vi "课堂.vi"() -> ()   [LabVIEW 2025]
panel:
  out "波形图表 7":dynamicdata(graph)
  out "波形图 4":cluster{dbl, dbl, dbl[]}[](graph)
  out "波形图表 6":dynamicdata(graph)
  out "波形图表 5":dbl[][](graph)
  out "波形图表 4":dbl[][](graph)
  out "波形图表 3":T1(graph)
  in  "数值":i32=40
  out "波形图表 2":dbl(graph)
  out "添加的数组":cluster{dbl[], dbl, dbl}[](array[cluster])
  out "波形图表":dbl[](graph)
  out "波形图 3":cluster{dbl[]}[](graph)
  out "波形图 2":dbl[][](graph)
  in  "采样点":i32=20
  out "波形图":dbl[](graph)=[0.8868508827682611, 0.2984304319078226, 0.11493741001008173, 0.9364201331616009, 0.9408037968299381, 0.6329733796655734, 0.6472915833351531, 0.9860727906146628, 0.3603313120178604, 0.38096386458152054, 0.8470946380077311, 0.620762260365446, 0.1766664398823562, 0.1967040576165764, 0.5080598419098434, 0.6274260346713301, 0.000348958293627355, 0.6443450592231559, 0.20809398466731732, 0.32035543006157274]
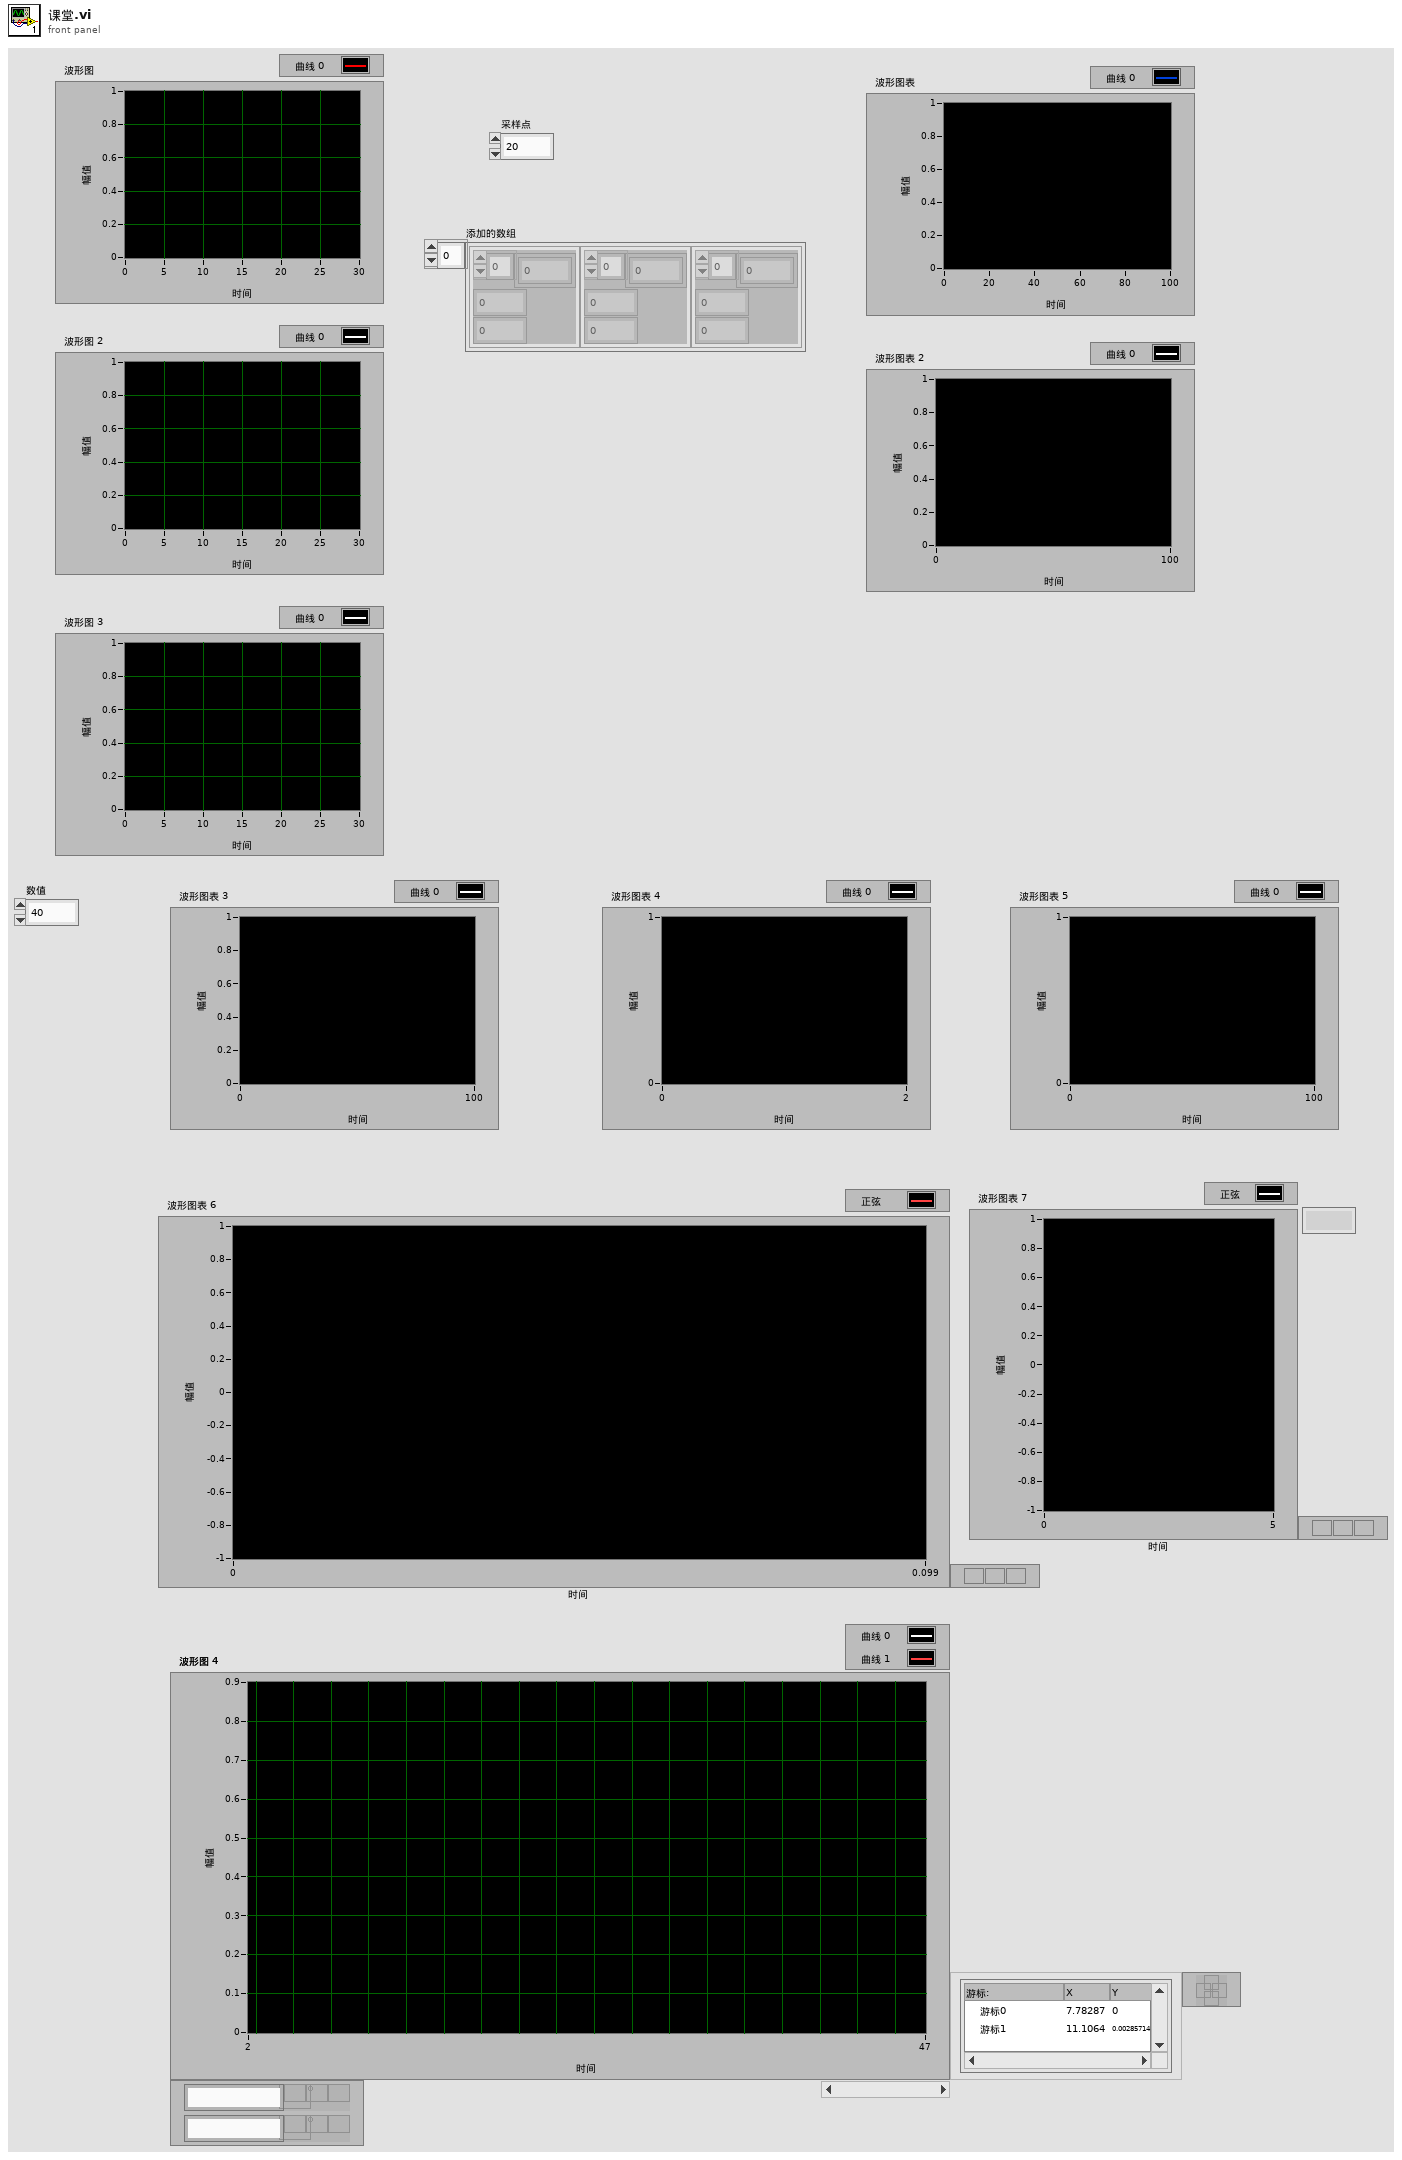
[diagram p1: front panel]
types:
  T1 = cluster{"number: 0 to 1":dbl, "number: 0 to 1":dbl}
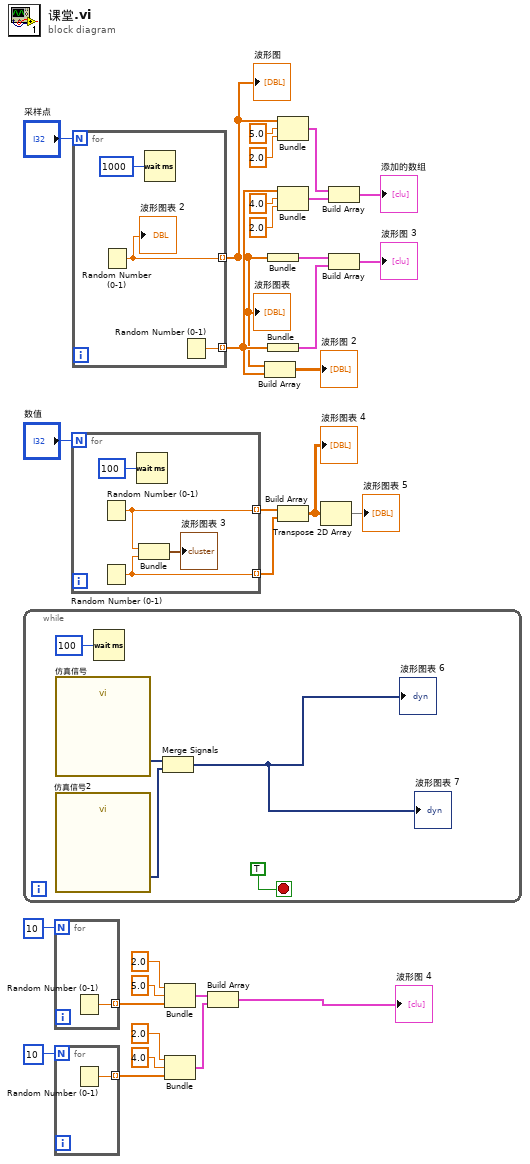
[diagram p0: block diagram]
diagram:
  n1 = while {
    stop <- TRUE stop-if-true
    n2 = call "仿真信号"() -> ("正弦"=w35:dynamicdata)  [unwired: 14 in, 1 out]
    n3 = call "仿真信号2"() -> ("正弦"=w34:dynamicdata)  [unwired: 14 in, 1 out]
    n4 = Wait (ms)(milliseconds to wait=u32 100 ("等待时间（毫秒）")) -> ()  [unwired: 1 out]
    n5 = Merge Signals(w35, w34) -> (→"波形图表 6" →"波形图表 7":dynamicdata)
  }
  n6 = for {
    N: 10 -> [_]
    tunnel: [w36] -> w4 mode=indexing
    n7 = Random Number (0-1)() -> (number: 0 to 1=w36:dbl)
  }
  n8 = for {
    N: 10 -> [_]
    tunnel: [w37] -> w2 mode=indexing
    n9 = Random Number (0-1)() -> (number: 0 to 1=w37:dbl)
  }
  n10 = for {
    N: "数值" -> [_]
    tunnel: [w39] -> w15 mode=indexing
    tunnel: [w38] -> w14 mode=indexing
    n11 = Random Number (0-1)() -> (number: 0 to 1=w39:dbl)
    n12 = Random Number (0-1)() -> (number: 0 to 1=w38:dbl)
    n13 = Wait (ms)(milliseconds to wait=u32 100 ("等待时间（毫秒）")) -> ()  [unwired: 1 out]
    n14 = Bundle("number: 0 to 1"=w39, "number: 0 to 1"=w38) -> (→"波形图表 3":T1)  [unwired: 1 in]
  }
  n15 = for {
    N: "采样点" -> [_]
    tunnel: [w43] -> w17 mode=indexing
    tunnel: [w44] -> w25 mode=indexing
    n16 = Random Number (0-1)() -> (number: 0 to 1=w43:dbl)
    "波形图表 2" <- w43
    n17 = Wait (ms)(milliseconds to wait=u32 1000 ("等待时间（毫秒）")) -> ()  [unwired: 1 out]
    n18 = Random Number (0-1)() -> (number: 0 to 1=w44:dbl)
  }
  "波形图" <- w17
  "波形图表" <- w17
  n19 = Bundle(2.0, 5.0, w4) -> (w7:cluster{dbl, dbl, dbl[]})  [unwired: 1 in]
  n20 = Bundle(2.0, 4.0, w2) -> (w6:cluster{dbl, dbl, dbl[]})  [unwired: 1 in]
  n21 = Build Array(w7, w6) -> (→"波形图 4":cluster{dbl, dbl, dbl[]}[])
  n22 = Build Array(w17, w25) -> (→"波形图 2":dbl[][])
  n23 = Bundle(w17) -> (w28:cluster{dbl[]})  [unwired: 1 in]
  n24 = Bundle(w25) -> (w27:cluster{dbl[]})  [unwired: 1 in]
  n25 = Bundle(w17, 5.0, 2.0) -> (w20:cluster{dbl[], dbl, dbl})  [unwired: 1 in]
  n26 = Bundle(w25, 4.0, 2.0) -> (w19:cluster{dbl[], dbl, dbl})  [unwired: 1 in]
  n27 = Build Array(w15, w14) -> (w13:dbl[][])
  "波形图表 4" <- w13
  n28 = Transpose 2D Array(2D array=w13) -> (transposed array=→"波形图表 5":dbl[][])
  n29 = Build Array(w20, w19) -> (→"添加的数组":cluster{dbl[], dbl, dbl}[])
  n30 = Build Array(w28, w27) -> (→"波形图 3":cluster{dbl[]}[])
